vi "顺序执行.vi"(1 "error in (no error)":errorcluster) -> (0 "error out":errorcluster)   [LabVIEW 2022 SP3]
doc: "本VI是为《我和LabVIEW》一书编写的示例。\n关于本书的介绍请参考网页：\nhttp://ruanqizhen.spaces.live.com/blog/cns!5852D4F797C53FB6!4310.entry"
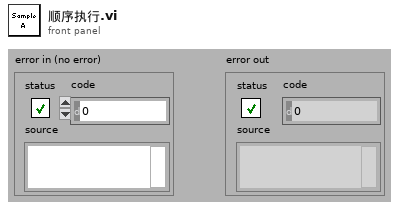
[diagram p1: front panel]
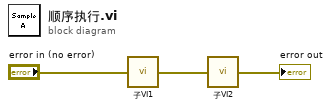
[diagram p0: block diagram]
diagram:
  n1 = call "子VI1.vi"("error in (no error)"="error in (no error)") -> ("error out"=w2:errorcluster)
  n2 = call "子VI2.vi"("error in (no error)"=w2) -> ("error out"=→"error out":errorcluster)
